vi "GetBufferFromFile.vi"(8 "Error IN":errorcluster caption="에러 입력", 10 "FilePath":path, 11 "HEKAdat.lvclass IN":refnum<class "HEKAdat.lvclass">) -> (0 "Error OUT":errorcluster caption="에러 출력", 2 "Buffer":string, 3 "HEKAdat.lvclass OUT":refnum<class "HEKAdat.lvclass">)   [LabVIEW 2017, in "HEKAdat.lvclass"]
uses:
  HEKAdat.lvclass
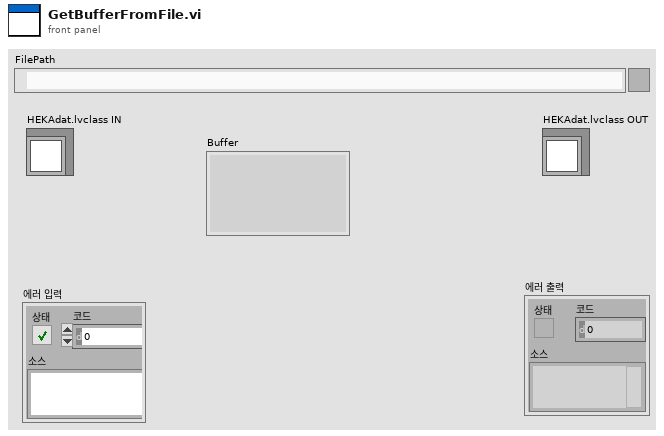
[diagram p1: front panel]
types:
  T1 = enum16{"open", "replace", "create", "open or create", "replace or create", "replace or create with confirmation"}
  T2 = enum16{"big-endian, network order", "native, host order", "little-endian"}
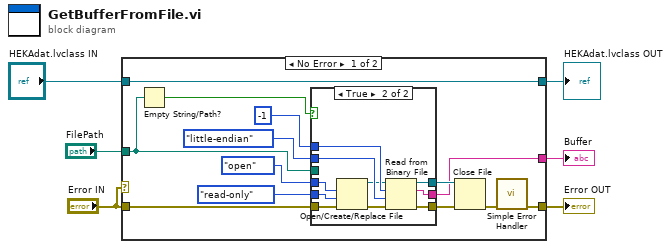
[diagram p0: block diagram]
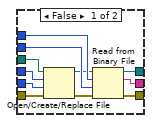
[diagram p2: hidden frame]
diagram:
  n1 = case shown="No Error" "Error IN" {
    tunnel: "Error IN" -> [w18 w41]
    tunnel: [w17 w41] -> w6
    tunnel: "HEKAdat.lvclass IN" -> [w15 w42]
    tunnel: [w15 w42] -> w4
    tunnel: "FilePath" -> [w14 _]
    tunnel: [w9 _] -> w1
    frame No Error {
      n2 = Empty String/Path?(string/path=w14) -> (empty?=w16:bool)
      n3 = case shown="True" w16 {
        tunnel: w18 -> [w21 w32]
        tunnel: w14 -> [w25 _]
        tunnel: [w30 w40] -> w13
        tunnel: [w29 w39] -> w12
        tunnel: -1 ("카운트(1)") -> [w28 w36]
        tunnel: T2."little-endian" ("바이트 순서(0:big-endian, network order)") -> [w27 w37]
        tunnel: [w26 w38] -> w9
        tunnel: T1."open" ("operation (0:open)") -> [w23 w34]
        tunnel: enum16{"read/write", "read-only", "write-only"}."read-only" ("access (0:read/write)") -> [w22 w33]
        frame False {
          n4 = Open/Create/Replace File(file path (use dialog)=w25, error in=w21, operation (0:open)=w23, access (0:read/write)=w22) -> (refnum out=w24:refnum<file>, error out=w20:errorcluster)  [unwired: 2 in, 1 out]
          n5 = Read from Binary File(8:w20, 9:w27, 10:w28, 11:w24) -> (0:w30:errorcluster, 2:w26:string, 3:w29:refnum<file>)  [unwired: 2 in, 1 out]
        }
        frame True {
          n6 = Open/Create/Replace File(error in=w32, operation (0:open)=w34, access (0:read/write)=w33) -> (refnum out=w35:refnum<file>, error out=w31:errorcluster)  [unwired: 3 in, 1 out]
          n7 = Read from Binary File(8:w31, 9:w37, 10:w36, 11:w35) -> (0:w40:errorcluster, 2:w38:string, 3:w39:refnum<file>)  [unwired: 2 in, 1 out]
        }
      }
      n8 = Close File(refnum=w12, error in=w13) -> (error out=w19:errorcluster)  [unwired: 1 out]
      n9 = call <vilib>:"Simple Error Handler.vi"("error in (no error)"=w19) -> ("error out"=w17:errorcluster)  [unwired: 4 in, 4 out]
    }
    frame Error {
    }
  }
  "Error OUT" <- w6
  "HEKAdat.lvclass OUT" <- w4
  "Buffer" <- w1
